vi "Mouse Zoom.vi"(7 "PlatMods":T1, 8 "error in (no error)":errorcluster, 9 "XY":cluster{"X":dbl, "Y":dbl}, 10 "Delta":i32, 11 "XY Graph":refnum<vi>) -> ()   [LabVIEW 2014, in "Graph Extensions.lvlib"]
doc: "Zooming works for several areas:\n\n1. No modifiers, just straight scroll wheel. This zooms on the X-Axis to zoom in and out\n2. SHIFT, changes the zoom to be on the Y-Axis\n3. CTRL, changes to a pan mode, sliding on the X-Axis with the scroll wheel\n4. CTRL SHIFT, pans on the Y-Axis with the scroll wheel"
uses:
  Graph Extensions.lvlib
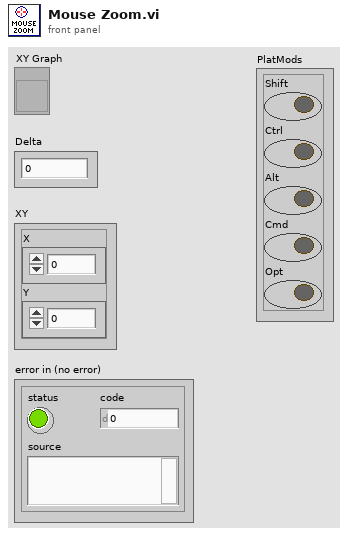
[diagram p1: front panel]
types:
  T1 = cluster{"Shift":bool, "Ctrl":bool, "Alt":bool, "Cmd":bool, "Opt":bool}
  T2 = typedef "LVRectTypeDef.ctl" = cluster{"Left":i16, "Top":i16, "Right":i16, "Bottom":i16}
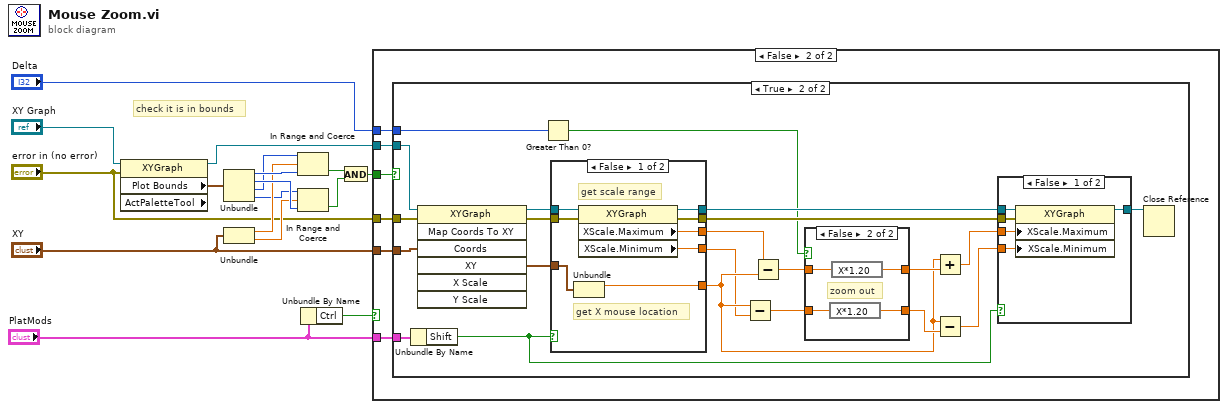
[diagram p0: block diagram]
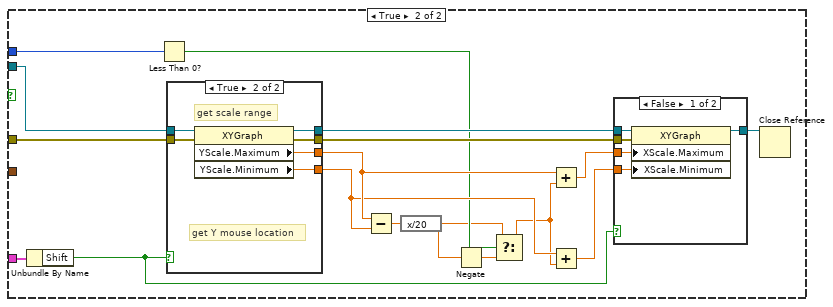
[diagram p3: hidden frame]
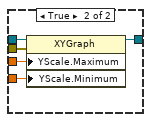
[diagram p4: hidden frame]
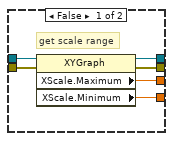
[diagram p5: hidden frame]
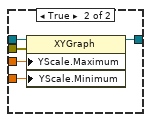
[diagram p7: hidden frame]
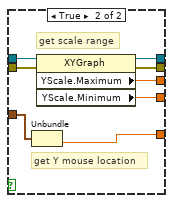
[diagram p8: hidden frame]
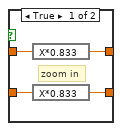
[diagram p9: hidden frame]
diagram:
  # "check it is in bounds"
  n1 = property on="Property Node" class="XYGraph" props=["Plot Bounds", "ActPaletteTool"](reference="XY Graph", error in="error in (no error)") -> (reference out=w3:refnum<vi>, "Plot Bounds"=w6:T2)  [unwired: 2 out]
  n2 = Unbundle(w6) -> ("Left"=w16:i16, "Top"=w15:i16, "Right"=w12:i16, "Bottom"=w11:i16)
  n3 = Unbundle("XY") -> ("X"=w13:dbl, "Y"=w14:dbl)
  n4 = In Range and Coerce(upper limit=w12, x=w13, lower limit=w16) -> (In Range?=w10:bool)  [unwired: 1 out]
  n5 = In Range and Coerce(upper limit=w11, x=w14, lower limit=w15) -> (In Range?=w9:bool)  [unwired: 1 out]
  n6 = Unbundle By Name("PlatMods") -> ("Ctrl"=w1:bool)
  n7 = And(x=w10, y=w9) -> (x .and. y?=w4:bool)
  n8 = case shown="False" w1 {
    tunnel: "Delta" -> [w23 w68]
    tunnel: "error in (no error)" -> [w22 w67]
    tunnel: "XY" -> [w21 w66]
    tunnel: w4 -> [w20 w65]
    tunnel: w3 -> [w19 w64]
    tunnel: "PlatMods" -> [w18 w63]
    frame True {
      # "Holding CTRL - PAN Left and Right"
      n9 = case shown="False" w20 {
        tunnel: w23 -> [_ w36]
        tunnel: w19 -> [_ w32]
        tunnel: w22 -> [_ w31]
        tunnel: w21 -> [_ _]
        tunnel: w18 -> [_ w34]
        frame False {
          # "not in the plot range, so ignore the scroll wheel"
        }
        frame True {
          n10 = Unbundle By Name(w34) -> ("Shift"=w33:bool)
          n11 = Less Than 0?(x=w36) -> (x < 0?=w27:bool)
          n12 = case shown="True" w33 {
            tunnel: [w56 w62] -> w29
            tunnel: [w55 w61] -> w28
            tunnel: [w54 w60] -> w38
            tunnel: [w53 w59] -> w37
            tunnel: w31 -> [w52 w58]
            tunnel: w32 -> [w51 w57]
            frame False {
              # "get scale range"
              n13 = property on="Property Node" class="XYGraph"(reference=w51, error in=w52) -> (reference out=w53:refnum<vi>, error out=w54:errorcluster, "XScale.Maximum"=w56:dbl, "XScale.Minimum"=w55:dbl)
            }
            frame True {
              # "get scale range"
              # "get Y mouse location"
              n14 = property on="Property Node" class="XYGraph"(reference=w57, error in=w58) -> (reference out=w59:refnum<vi>, error out=w60:errorcluster, "YScale.Maximum"=w62:dbl, "YScale.Minimum"=w61:dbl)
            }
          }
          n15 = Subtract(x=w29, y=w28) -> (x-y=w30:dbl)
          n16 = expression code="x/20"(w30) -> (w24:dbl)
          n17 = Negate(x=w24) -> (-x=w26:dbl)
          n18 = Select(t=w24, s=w27, f=w26) -> (s? t:f=w25:dbl)
          n19 = Add(x=w29, y=w25) -> (x+y=w39:dbl)
          n20 = Add(x=w28, y=w25) -> (x+y=w40:dbl)
          n21 = case shown="False" w33 {
            tunnel: w40 -> [w41 w50]
            tunnel: w39 -> [w42 w49]
            tunnel: w38 -> [w44 w48]
            tunnel: w37 -> [w45 w47]
            tunnel: [w43 w46] -> w35
            frame False {
              n22 = property on="Property Node" class="XYGraph"(reference=w45, error in=w44, "XScale.Maximum"=w42, "XScale.Minimum"=w41) -> (reference out=w43:refnum<vi>)  [unwired: 1 out]
            }
            frame True {
              n23 = property on="Property Node" class="XYGraph"(reference=w47, error in=w48, "YScale.Maximum"=w49, "YScale.Minimum"=w50) -> (reference out=w46:refnum<vi>)  [unwired: 1 out]
            }
          }
          n24 = Close Reference(reference=w35) -> ()  [unwired: 1 in, 1 out]
        }
      }
    }
    frame False {
      n25 = case shown="True" w65 {
        tunnel: w68 -> [_ w86]
        tunnel: w64 -> [_ w80]
        tunnel: w67 -> [_ w79]
        tunnel: w66 -> [_ w78]
        tunnel: w63 -> [_ w77]
        frame False {
          # "not in the plot range, so ignore the scroll wheel"
        }
        frame True {
          n26 = Unbundle By Name(w77) -> ("Shift"=w76:bool)
          n27 = invoke on="Invoke Node" class="XYGraph" method="Map Coords To XY"(reference=w80, error in=w79, "Coords"=w78) -> (reference out=w82:refnum<vi>, error out=w83:errorcluster, "XY"=w84:cluster{"X":dbl, "Y":dbl})  [unwired: 4 in, 4 out]
          n28 = Greater Than 0?(x=w86) -> (x > 0?=w85:bool)
          n29 = case shown="False" w76 {
            tunnel: [w108 w116] -> w73
            tunnel: [w107 w115] -> w70
            tunnel: [w106 w109] -> w71
            tunnel: [w105 w114] -> w88
            tunnel: [w104 w113] -> w87
            tunnel: w84 -> [w103 w112]
            tunnel: w83 -> [w102 w111]
            tunnel: w82 -> [w101 w110]
            frame False {
              # "get scale range"
              # "get X mouse location"
              n30 = Unbundle(w103) -> ("X"=w106:dbl)  [unwired: 1 out]
              n31 = property on="Property Node" class="XYGraph"(reference=w101, error in=w102) -> (reference out=w104:refnum<vi>, error out=w105:errorcluster, "XScale.Maximum"=w108:dbl, "XScale.Minimum"=w107:dbl)
            }
            frame True {
              # "get scale range"
              # "get Y mouse location"
              n32 = Unbundle(w112) -> ("Y"=w109:dbl)  [unwired: 1 out]
              n33 = property on="Property Node" class="XYGraph"(reference=w110, error in=w111) -> (reference out=w113:refnum<vi>, error out=w114:errorcluster, "YScale.Maximum"=w116:dbl, "YScale.Minimum"=w115:dbl)
            }
          }
          n34 = Subtract(x=w71, y=w70) -> (x-y=w69:dbl)
          n35 = Subtract(x=w73, y=w71) -> (x-y=w72:dbl)
          n36 = case shown="False" w85 {
            tunnel: w72 -> [w120 w124]
            tunnel: [w119 w123] -> w89
            tunnel: w69 -> [w118 w122]
            tunnel: [w117 w121] -> w75
            frame True {
              # "zoom in"
              n37 = expression code="X*0.833"(w120) -> (w119:dbl)
              n38 = expression code="X*0.833"(w118) -> (w117:dbl)
            }
            frame False {
              # "zoom out"
              n39 = expression code="X*1.20"(w122) -> (w121:dbl)
              n40 = expression code="X*1.20"(w124) -> (w123:dbl)
            }
          }
          n41 = Add(x=w71, y=w89) -> (x+y=w90:dbl)
          n42 = Subtract(x=w71, y=w75) -> (x-y=w74:dbl)
          n43 = case shown="False" w76 {
            tunnel: w74 -> [w91 w100]
            tunnel: w90 -> [w92 w99]
            tunnel: w88 -> [w94 w98]
            tunnel: w87 -> [w95 w97]
            tunnel: [w93 w96] -> w81
            frame False {
              n44 = property on="Property Node" class="XYGraph"(reference=w95, error in=w94, "XScale.Maximum"=w92, "XScale.Minimum"=w91) -> (reference out=w93:refnum<vi>)  [unwired: 1 out]
            }
            frame True {
              n45 = property on="Property Node" class="XYGraph"(reference=w97, error in=w98, "YScale.Maximum"=w99, "YScale.Minimum"=w100) -> (reference out=w96:refnum<vi>)  [unwired: 1 out]
            }
          }
          n46 = Close Reference(reference=w81) -> ()  [unwired: 1 in, 1 out]
        }
      }
    }
  }
